vi "SignalTest.vi"() -> ()   [LabVIEW 2011]
uses:
  Signal.ctl
panel:
  in  "SW":bool
  out "Waveform Chart":i16(graph)
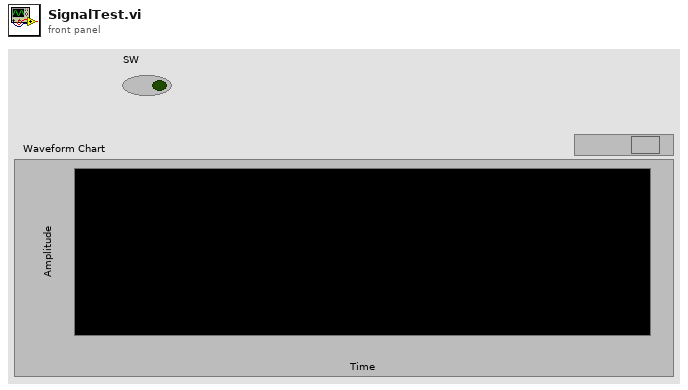
[diagram p1: front panel]
types:
  T1 = typedef "Signal.ctl" = enum16{"SIGFIRE", "SIGSTOPSCRIPT", "SIGSTARTGUN", "SIGSTOPGUN", "SIGDISABLED", "SIGENABLED", "SIGUDPTIMEOUT", "SIGNEWVISION_REMOTE", "SIGNEWVISION_LOCAL"}
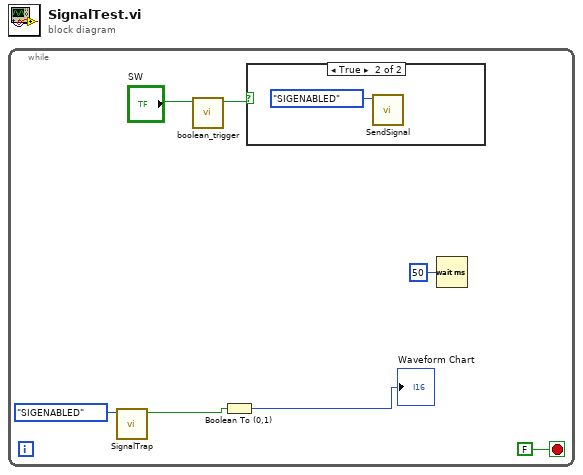
[diagram p0: block diagram]
diagram:
  n1 = while {
    stop <- FALSE stop-if-true
    n2 = call "SignalTrap.vi"("Signal"=Signal."SIGENABLED") -> ("Trapped Signal"=w4:bool)  [unwired: 10 in]
    n3 = call "boolean_trigger.vi"("Input"="SW") -> ("Rising Edge"=w6:bool)  [unwired: 10 in]
    n4 = Boolean To (0,1)(Boolean=w4) -> (0, 1=→"Waveform Chart":i16)
    n5 = case shown="True" w6 {
      frame False {
      }
      frame True {
        n6 = call "SendSignal.vi"("Signal"=Signal."SIGENABLED") -> ()  [unwired: 11 in]
      }
    }
    n7 = Wait (ms)(milliseconds to wait=u32 50) -> ()  [unwired: 1 out]
  }
